vi "Choreo_Choreo_SwerveControllerPackConfig.vi"(0 "X Y Vel Tolerance M/S":dbl=1.0, 1 "Rot Vel Tolerance Deg/S":dbl=30.0, 4 "Rot Tolerance Deg":dbl=10.0, 5 "X_Adv PID Limits":T1={"MaxInput"=0.0, "MinInput"=0.0, "Continuous"=FALSE, "MaxOutput"=9.9e+32, "MinOutput"=-9.9e+32}, 6 "X Y Pos Tolerance M":dbl=0.0381, 7 "X_Adv PID Tuning":T2={"Kf"=1.0, "Kp"=3.0, "Ki"=0.0, "Kd"=0.0, "MaximumIntegral"=9.9e+30, "MinimumIntegral"=-9.9e+30, "Filter Derivative"=FALSE}, 8 "Rot_Adv PID Tuning":T2={"Kf"=1.0, "Kp"=5.0, "Ki"=0.0, "Kd"=0.0, "MaximumIntegral"=9.9e+30, "MinimumIntegral"=-9.9e+30, "Filter Derivative"=FALSE}, 9 "Rot_Adv PID Limits":T1={"MaxInput"=3.141592653589793, "MinInput"=-3.141592653589793, "Continuous"=TRUE, "MaxOutput"=9.9e+32, "MinOutput"=-9.9e+32}, 10 "Y_Adv PID Tuning":T2={"Kf"=1.0, "Kp"=4.0, "Ki"=0.0, "Kd"=0.0, "MaximumIntegral"=9.9e+30, "MinimumIntegral"=-9.9e+30, "Filter Derivative"=FALSE}, 11 "Y_Adv PID Limits":T1={"MaxInput"=0.0, "MinInput"=0.0, "Continuous"=FALSE, "MaxOutput"=9.9e+32, "MinOutput"=-9.9e+32}) -> (3 "ChoreoSwerveControlConfig":T3={"X_Adv PID Tuning"={"Kf"=0.0, "Kp"=3.0, "Ki"=0.0, "Kd"=0.0, "MaximumIntegral"=9.9e+30, "MinimumIntegral"=-9.9e+30, "Filter Derivative"=FALSE}, "X_Adv PID Limits"={"MaxInput"=0.0, "MinInput"=0.0, "Continuous"=FALSE, "MaxOutput"=9.9e+32, "MinOutput"=-9.9e+32}, "Y_Adv PID Tuning"={"Kf"=0.0, "Kp"=4.0, "Ki"=0.0, "Kd"=0.0, "MaximumIntegral"=9.9e+30, "MinimumIntegral"=-9.9e+30, "Filter Derivative"=FALSE}, "Y_Adv PID Limits"={"MaxInput"=0.0, "MinInput"=0.0, "Continuous"=FALSE, "MaxOutput"=9.9e+32, "MinOutput"=-9.9e+32}, "Rot_Adv PID Tuning"={"Kf"=0.0, "Kp"=5.0, "Ki"=0.0, "Kd"=0.0, "MaximumIntegral"=9.9e+30, "MinimumIntegral"=-9.9e+30, "Filter Derivative"=FALSE}, "Rot_Adv PID Limits"={"MaxInput"=3.141592653589793, "MinInput"=-3.14159, "Continuous"=TRUE, "MaxOutput"=9.9e+32, "MinOutput"=-9.9e+32}, "X Y Pos Tolerance M"=0.0381, "Rot Tolerance Deg"=0.0523599, "X Y Vel Tolerance M/S"=1.0, "Rot Vel Tolerance Deg/S"=20.0})   [LabVIEW 2019, in "ChoreoLib.lvlib"]
doc: "Packs the configuration information for a Choreo Swerve Controller into a cluster for use by the Choreo Swerve Controller or the Choreo Swerve Command functions.\n\nNote:\n - Defaults have been chosen for the inputs, however tuning based on actual performance is advised.\n\nInputs:\n - X Adv PID Limits - cluster - Input and output limits for the X position PID (Optional.)\n - X Adv PID Tuning - cluster - Tuning values for the X position PID (optional)\n - Y Adv PID Limits - cluster - Input and output limits for the Y position PID (Optional.)\n - Y Adv PID Tuning - cluster - Tuning values for the Y position PID (optional)\n - Rot Adv PID Limits - cluster - Input and output limits for the rotation position PID. Note this PID must be set to continuous (Optional.)\n - Rot Adv PID Tuning - cluster - Tuning values for the rotational position PID (optional)\n - X Y Pos Tolerance - double - Distance (Meters) to be considered on target. (Defaultt 0.0381)\n - Rot Pos Tolerance - double - Rotation (Degrees) to be considered on target. (Defaultt 10.0)\n - X Y Vel Tolerance - double - Velocity (Meters/Second) to be considered on target. (Defaultt 1.0)\n - Rot Vel Tolerance - double - Velocity (Degrees/Second) to be considered on target. (Defaultt 30.0)\n\nOutputs:\n - ChoreoSwerveControlConfig - cluster - packed controller configuration."
uses:
  ChoreoLib.lvlib
  TypeDef/ChoreoSwerveControlConfig.ctl
  <vilib>/Rock Robotics/WPI/ThirdParty/JAS_Junk/TrajLib/TypeDef/PID_ADV_TUNING.ctl
  <vilib>/Rock Robotics/WPI/ThirdParty/JAS_Junk/TrajLib/TypeDef/PID_ADV_LIMITS.ctl
  <vilib>/Rock Robotics/WPI/ThirdParty/JAS_Junk/TrajLib/Trajectory_Library.lvlib
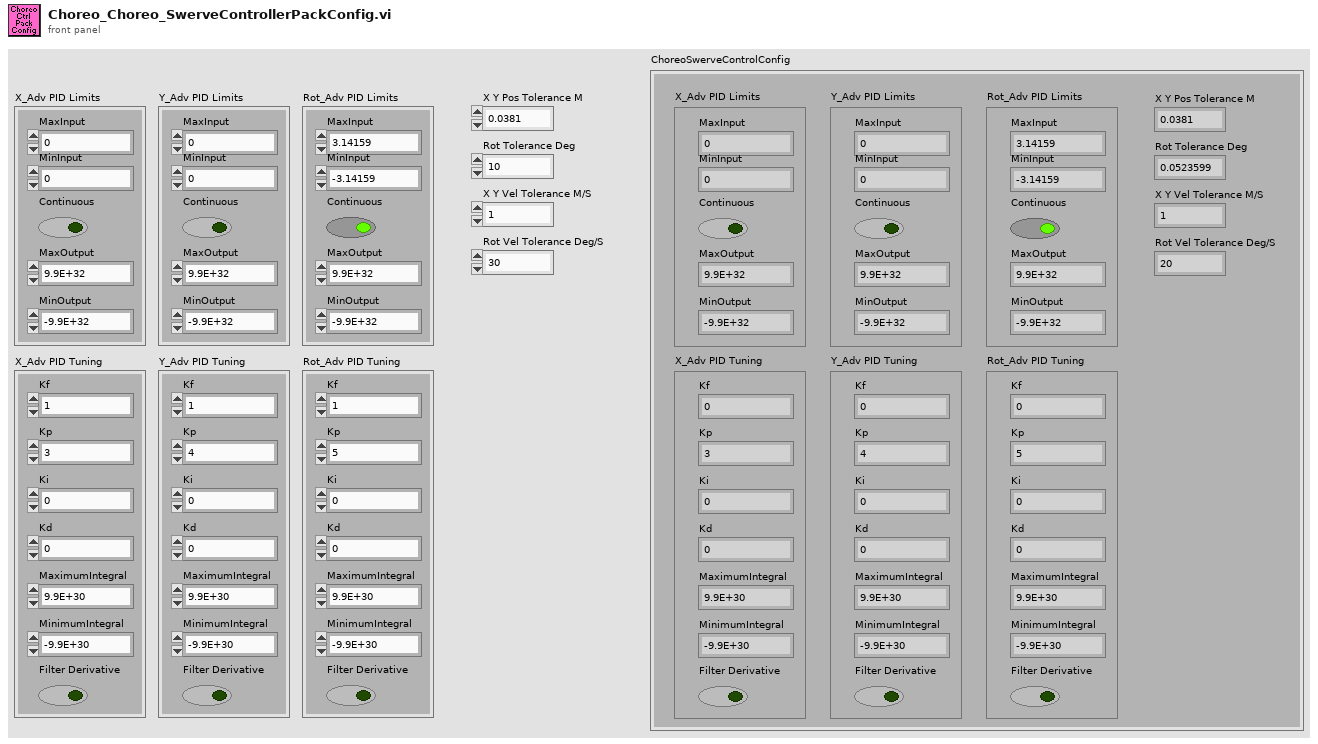
[diagram p1: front panel]
types:
  T1 = typedef "Trajectory_Library.lvlib/PID_ADV_LIMITS.ctl" = cluster{"MaxInput":dbl, "MinInput":dbl, "Continuous":bool, "MaxOutput":dbl, "MinOutput":dbl}
  T2 = typedef "Trajectory_Library.lvlib/PID_ADV_TUNING.ctl" = cluster{"Kf":dbl, "Kp":dbl, "Ki":dbl, "Kd":dbl, "MaximumIntegral":dbl, "MinimumIntegral":dbl, "Filter Derivative":bool}
  T3 = typedef "ChoreoLib.lvlib/ChoreoSwerveControlConfig.ctl" = cluster{"X_Adv PID Tuning":T2, "X_Adv PID Limits":T1, "Y_Adv PID Tuning":T2, "Y_Adv PID Limits":T1, "Rot_Adv PID Tuning":T2, "Rot_Adv PID Limits":T1, "X Y Pos Tolerance M":dbl, "Rot Tolerance Deg":dbl, "X Y Vel Tolerance M/S":dbl, "Rot Vel Tolerance Deg/S":dbl}
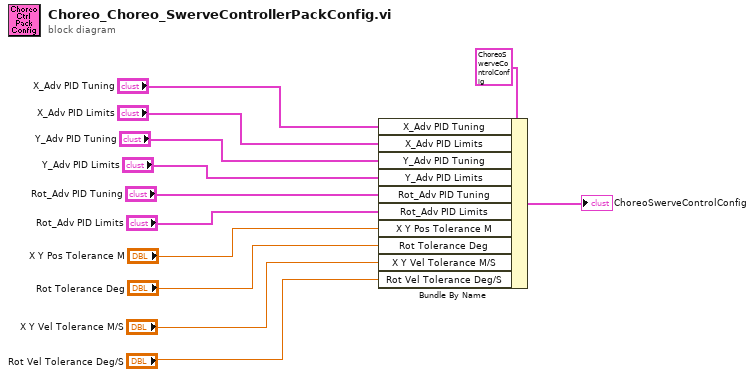
[diagram p0: block diagram]
diagram:
  n1 = Bundle By Name(cluster=T3 {"X_Adv PID Tuning"={"Kf"=0.0, "Kp"=3.0, "Ki"=0.0, "Kd"=0.0, "MaximumIntegral"=9.9e+30, "MinimumIntegral"=-9.9e+30, "Filter Derivative"=FALSE}, "X_Adv PID Limits"={"MaxInput"=0.0, "MinInput"=0.0, "Continuous"=FALSE, "MaxOutput"=9.9e+32, "MinOutput"=-9.9e+32}, "Y_Adv PID Tuning"={"Kf"=0.0, "Kp"=4.0, "Ki"=0.0, "Kd"=0.0, "MaximumIntegral"=9.9e+30, "MinimumIntegral"=-9.9e+30, "Filter Derivative"=FALSE}, "Y_Adv PID Limits"={"MaxInput"=0.0, "MinInput"=0.0, "Continuous"=FALSE, "MaxOutput"=9.9e+32, "MinOutput"=-9.9e+32}, "Rot_Adv PID Tuning"={"Kf"=0.0, "Kp"=5.0, "Ki"=0.0, "Kd"=0.0, "MaximumIntegral"=9.9e+30, "MinimumIntegral"=-9.9e+30, "Filter Derivative"=FALSE}, "Rot_Adv PID Limits"={"MaxInput"=3.141592653589793, "MinInput"=-3.14159, "Continuous"=TRUE, "MaxOutput"=9.9e+32, "MinOutput"=-9.9e+32}, "X Y Pos Tolerance M"=0.0381, "Rot Tolerance Deg"=0.0523599, "X Y Vel Tolerance M/S"=1.0, "Rot Vel Tolerance Deg/S"=20.0} ("ChoreoSwerveControlConfig"), "X_Adv PID Tuning"="X_Adv PID Tuning", "X_Adv PID Limits"="X_Adv PID Limits", "Y_Adv PID Tuning"="Y_Adv PID Tuning", "Y_Adv PID Limits"="Y_Adv PID Limits", "Rot_Adv PID Tuning"="Rot_Adv PID Tuning", "Rot_Adv PID Limits"="Rot_Adv PID Limits", "X Y Pos Tolerance M"="X Y Pos Tolerance M", "Rot Tolerance Deg"="Rot Tolerance Deg", "X Y Vel Tolerance M/S"="X Y Vel Tolerance M/S", "Rot Vel Tolerance Deg/S"="Rot Vel Tolerance Deg/S") -> (→"ChoreoSwerveControlConfig":T3)
